vi "SetPanesColors.vi"(8 "error in (no error)":errorcluster, 10 "Panes":T2, 11 "Colors":T1={"Top Color"=16448250, "Left Color"=16448250, "Center Color"=16448250, "Right Color"=16448250, "Bottom Color"=16448250}) -> (0 "error out":errorcluster)   [LabVIEW 2022 SP3, in "PentaPanesLibrary.lvlib" / "PentaPanes.lvclass"]
uses:
  PentaPanes.lvclass
  PanesCluster.ctl
  PanesColors.ctl
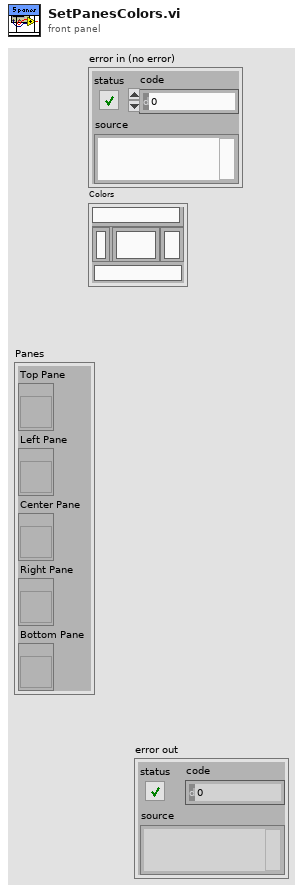
[diagram p1: front panel]
types:
  T1 = typedef "PentaPanesLibrary.lvlib/PentaPanes.lvclass/PanesColors.ctl" = cluster{"Top Color":u32, "Left Color":u32, "Center Color":u32, "Right Color":u32, "Bottom Color":u32}
  T2 = typedef "PentaPanesLibrary.lvlib/PentaPanes.lvclass/PanesCluster.ctl" = cluster{"Top Pane":refnum<vi>, "Left Pane":refnum<vi>, "Center Pane":refnum<vi>, "Right Pane":refnum<vi>, "Bottom Pane":refnum<vi>}
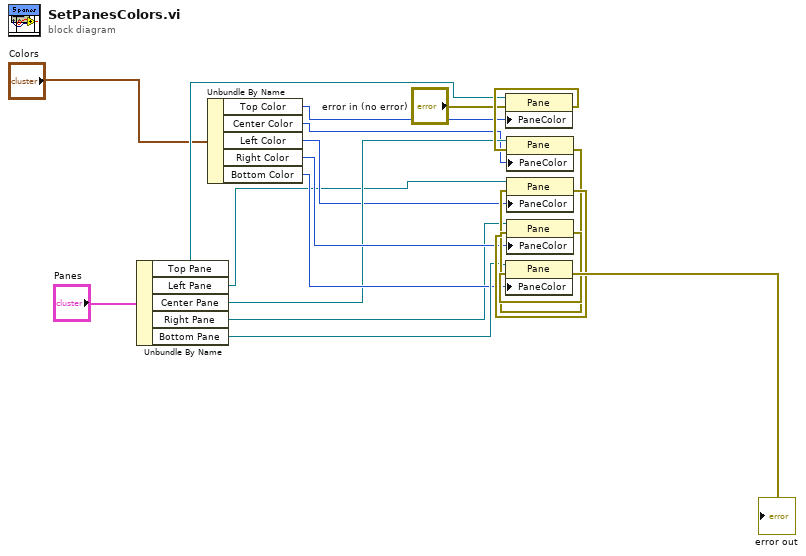
[diagram p0: block diagram]
diagram:
  n1 = Unbundle By Name("Panes") -> ("Top Pane"=w3:refnum<vi>, "Left Pane"=w2:refnum<vi>, "Center Pane"=w9:refnum<vi>, "Right Pane"=w10:refnum<vi>, "Bottom Pane"=w13:refnum<vi>)
  n2 = Unbundle By Name("Colors") -> ("Top Color"=w6:u32, "Center Color"=w7:u32, "Left Color"=w8:u32, "Right Color"=w11:u32, "Bottom Color"=w12:u32)
  n3 = property class="Pane"(reference=w3, error in="error in (no error)", "PaneColor"=w6) -> (error out=w14:errorcluster)  [unwired: 1 out]
  n4 = property class="Pane"(reference=w9, error in=w14, "PaneColor"=w7) -> (error out=w15:errorcluster)  [unwired: 1 out]
  n5 = property class="Pane"(reference=w2, error in=w15, "PaneColor"=w8) -> (error out=w16:errorcluster)  [unwired: 1 out]
  n6 = property class="Pane"(reference=w10, error in=w16, "PaneColor"=w11) -> (error out=w17:errorcluster)  [unwired: 1 out]
  n7 = property class="Pane"(reference=w13, error in=w17, "PaneColor"=w12) -> (error out=→"error out":errorcluster)  [unwired: 1 out]
